vi "GetControlStyles.vi"(11 "Control Styles Path":path) -> (3 "constructors":variant)   [LabVIEW 2014, in "PythonConverter_GUI.lvclass"]
uses:
  PythonConverter_GUI.lvclass
  TypeDefs/ConstructorInfo.ctl
  <vilib>/Utility/file.llb/Read From Spreadsheet File (string).vi
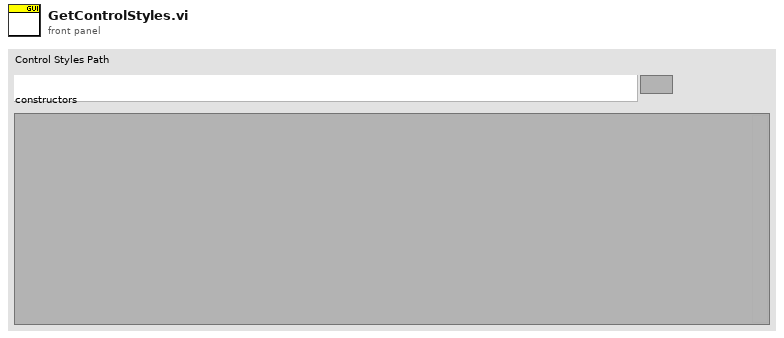
[diagram p1: front panel]
types:
  T1 = typedef "PythonConverter_GUI.lvclass/ConstructorInfo.ctl" = cluster{"Style ID":u32, "python class":string, "python module":string, "python module name":string, "check datatype":bool, "get image":bool}
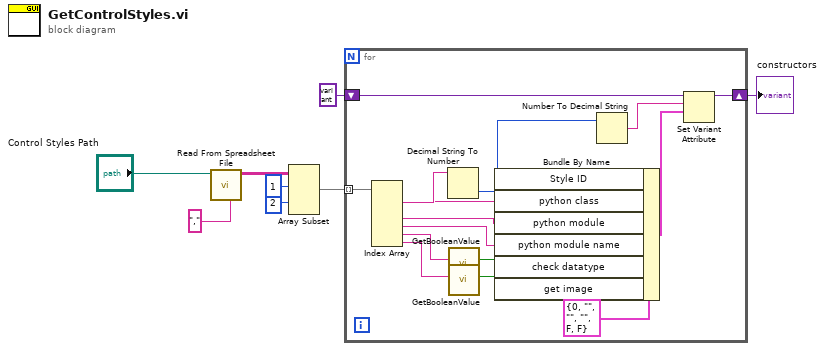
[diagram p0: block diagram]
diagram:
  n1 = call-poly <vilib>:"Read From Spreadsheet File.vi"("delimiter (\\t)"="," ("delimiter (\\t)"), "file path (dialog if empty)"="Control Styles Path") -> ("all rows"=w6:string[][])  [unwired: 5 in, 4 out]
  n2 = Array Subset(array=w6, index (row)=1 ("index"), index (col)=2 ("index")) -> (w4:string[][])  [unwired: 2 in]
  n3 = for {
    tunnel: w4 -> [w23] mode=indexing
    shift-right: [w13] -> w1
    shift-left: variant -> [w10]
    n4 = Index Array(array=w23) -> (element #1=w22:string, element #2=w20:string, element #3=w19:string, element #4=w18:string, element #5=w14:string, element #6=w17:string)  [unwired: 6 in]
    n5 = Decimal String To Number(string=w22) -> (number=w12:i32)  [unwired: 2 in, 1 out]
    n6 = call "GetBooleanValue.vi"("true/false string"=w14) -> ("value"=w15:bool)  [unwired: 10 in]
    n7 = call "GetBooleanValue.vi"("true/false string"=w17) -> ("value"=w16:bool)  [unwired: 10 in]
    n8 = Bundle By Name(cluster=T1 {"Style ID"=0, "python class"="", "python module"="", "python module name"="", "check datatype"=FALSE, "get image"=FALSE} ("Constructor Info"), "Style ID"=w12, "python class"=w20, "python module"=w19, "python module name"=w18, "check datatype"=w15, "get image"=w16) -> (w9:T1)
    n9 = Number To Decimal String(number=w12) -> (decimal integer string=w11:string)  [unwired: 1 in]
    n10 = Set Variant Attribute(Variant=w10, name=w11, value=w9) -> (Variant out=w13:variant)  [unwired: 1 in, 2 out]
  }
  "constructors" <- w1
